vi "Generator sygnałów testowych.vi"(2 "częstotliwość\nakwizycji próbek":dbl=10000.0 format="%.2f", 3 "liczba punktów\n      (1024)":i32=1024, 4 "amplituda szumów":dbl format="%.2f", 5 "amplituda sygnału":dbl format="%.2f", 6 "częstotliwość\n   sygnału":dbl(slide) scale=50.0..200.0, 7 "rodzaj sygnału":u16(ring) items=["szum", "zewnętrzny", "sinus", "prostokąt", "trójkąt"]) -> (0 "czas akwizycji\n      próbek":dbl=0.000125 format="%.2e", 1 "sygnał wyjściowy":dbl[](array[numeric]) format="%.2f")   [LabVIEW 2020]
uses:
  <vilib>/Analysis/NI_AALBase.lvlib
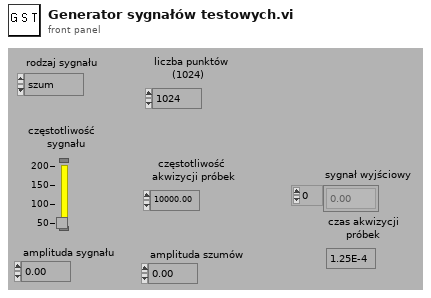
[diagram p1: front panel]
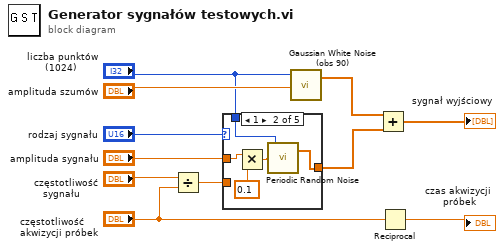
[diagram p0: block diagram]
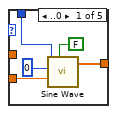
[diagram p2: hidden frame]
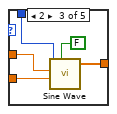
[diagram p3: hidden frame]
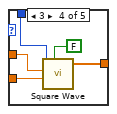
[diagram p4: hidden frame]
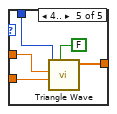
[diagram p5: hidden frame]
diagram:
  n1 = Divide(x="częstotliwość\n   sygnału", y="częstotliwość\nakwizycji próbek") -> (x/y=w11:dbl)
  n2 = case shown="1" "rodzaj sygnału" {
    tunnel: w11 -> [w16 _ w26 w31 w36]
    tunnel: "liczba punktów\n      (1024)" -> [w15 w20 w23 w30 w35]
    tunnel: [w13 w19 w24 w28 w33] -> w3
    tunnel: "amplituda sygnału" -> [_ w21 w22 w27 w32]
    frame ..0 {
      n3 = call <vilib>:"Sine Wave.vi"("samples"=w15, "amplitude"=u8 0, "frequency"=w16, "reset phase"=FALSE) -> ("sine wave"=w13:dbl[])  [unwired: 1 in, 2 out]
    }
    frame 1 {
      n4 = Multiply(x=w21, y=0.1) -> (x*y=w18:dbl)
      n5 = call <vilib>:"Periodic Random Noise.vi"("spectral amplitude"=w18, "samples"=w20) -> ("periodic random noise"=w19:dbl[])  [unwired: 1 in, 1 out]
    }
    frame 2 {
      n6 = call <vilib>:"Sine Wave.vi"("samples"=w23, "amplitude"=w22, "frequency"=w26, "reset phase"=FALSE) -> ("sine wave"=w24:dbl[])  [unwired: 1 in, 2 out]
    }
    frame 3 {
      n7 = call <vilib>:"Square Wave.vi"("samples"=w30, "reset phase"=FALSE, "amplitude"=w27, "frequency"=w31) -> ("square wave"=w28:dbl[])  [unwired: 2 in, 2 out]
    }
    frame 4.. {
      n8 = call <vilib>:"Triangle Wave.vi"("samples"=w35, "amplitude"=w32, "frequency"=w36, "reset phase"=FALSE) -> ("triangle wave"=w33:dbl[])  [unwired: 1 in, 2 out]
    }
  }
  n9 = call <vilib>:"Gaussian White Noise (obs 90).vi"("standard deviation"="amplituda szumów", "samples"="liczba punktów\n      (1024)") -> ("Gaussian noise pattern"=w2:dbl[])  [unwired: 1 in, 1 out]
  n10 = Add(x=w2, y=w3) -> (x+y=→"sygnał wyjściowy":dbl[])
  n11 = Reciprocal(x="częstotliwość\nakwizycji próbek") -> (1/x=→"czas akwizycji\n      próbek":dbl)
